vi "offset.to_json.vi"(8 "error in":errorcluster, 10 "offset":T1) -> (0 "error out":errorcluster, 2 "json":string)   [LabVIEW 2020, in "dataScopes.lvlib"]
uses:
  dataScopes.lvlib
  ab7c0d24-36bc-4d84-84a5-6341875158a7.vi
  offset.ctl
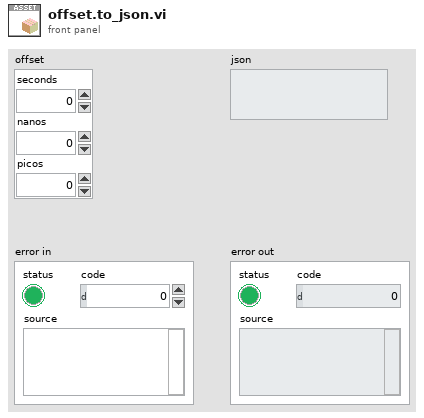
[diagram p1: front panel]
types:
  T1 = typedef "dataScopes.lvlib/offset.ctl" = cluster{"seconds":i32, "nanos":i32, "picos":i32}
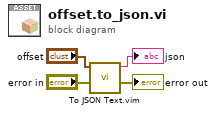
[diagram p0: block diagram]
diagram:
  n1 = call "To JSON Text.vim"("error in (no error)"="error in", "Anything"="offset") -> ("error out"=→"error out":errorcluster, "<JSON>"=→"json":string)  [unwired: 8 in]
